vi "Com_SECS Equipment _SECS Packet Write.vi"(8 "error in":errorcluster, 9 "Timeout":i32=1000, 10 "SECS Packet":T1, 11 "Buffer Data In":T5) -> (0 "error out":errorcluster, 3 "Buffer Data Out":T5)   [LabVIEW 2016]
uses:
  Data Def/Com_SECS Equipment _Buffer Data.ctl
  Data Def/Com_SECS Equipment _Connection Setting.ctl
  Data Def/Com_SECS Equipment _Timeout Setting.ctl
  Data Def/Com_SECS Equipment _SECS Packet.ctl
  Data Def/Com_SECS Equipment _Message Type.ctl
  Data Def/Com_SECS Equipment _Protocol Type.ctl
  Data Def/Com_SECS Equipment _Stream Type.ctl
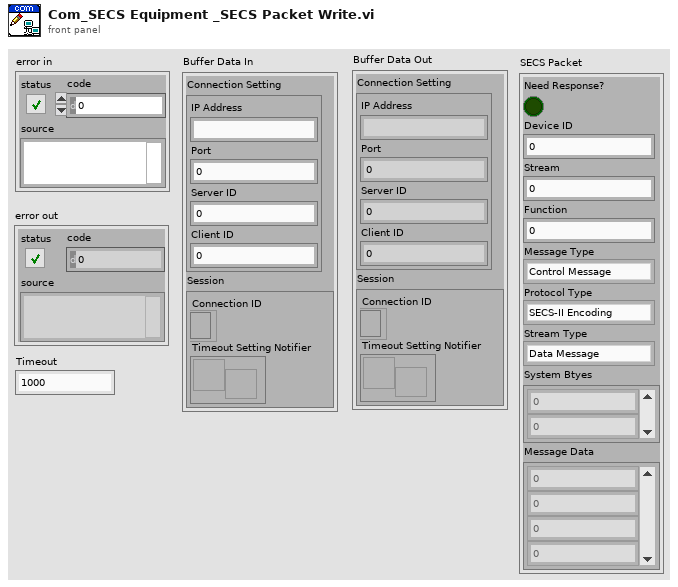
[diagram p1: front panel]
types:
  T1 = typedef "Com_SECS Equipment _SECS Packet.ctl" = cluster{"Need Response?":bool, "Device ID":u16, "Stream":u8, "Function":u8, "Message Type":T2, "Protocol Type":T3, "Stream Type":T4, "System Btyes":u8[], "Message Data":u8[]}
  T2 = typedef "Com_SECS Equipment _Message Type.ctl" = enum16{"Control Message", "Data Message"}
  T3 = typedef "Com_SECS Equipment _Protocol Type.ctl" = enum16{"SECS-II Encoding", "Reserved"}
  T4 = typedef "Com_SECS Equipment _Stream Type.ctl" = enum16{"Data Message", "Select.req", "Select.rsp", "Deselect.req", "Deselect.rsp", "Linktest.req", "Linktest.rsp", "Reject.req", "Separate.req", "Reserve"}
  T5 = typedef "Com_SECS Equipment _Buffer Data.ctl" = cluster{"Connection Setting":T6, "Session":cluster{"Connection ID":refnum<k5>, "Timeout Setting Notifier":refnum<notifier>}}
  T6 = typedef "Com_SECS Equipment _Connection Setting.ctl" = cluster{"IP Address":string, "Port":u16, "Server ID":u16, "Client ID":u16}
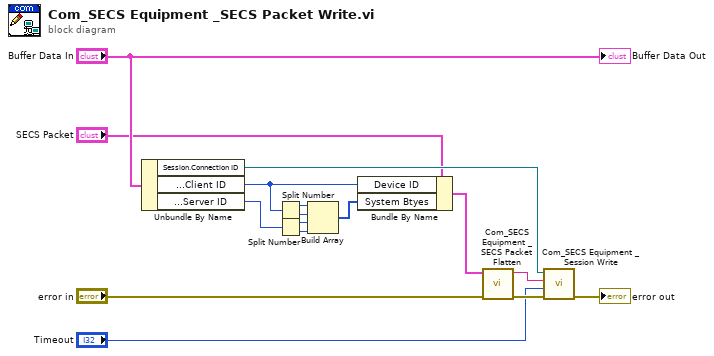
[diagram p0: block diagram]
diagram:
  n1 = Unbundle By Name("Buffer Data In") -> ("Session.Connection ID"=w3:refnum<k5>, "Connection Setting.Client ID"=w11:u16, "Connection Setting.Server ID"=w10:u16)
  n2 = Split Number(x=w11) -> (hi(x)=w9:u8, lo(x)=w8:u8)
  n3 = Split Number(x=w10) -> (hi(x)=w7:u8, lo(x)=w6:u8)
  n4 = Build Array(w9, w8, w7, w6) -> (w5:u8[])
  n5 = Bundle By Name(cluster="SECS Packet", "Device ID"=w11, "System Btyes"=w5) -> (w1:T1)
  n6 = call "Com_SECS Equipment _SECS Packet Flatten.vi"("error in"="error in", "SECS Packet"=w1) -> ("error out"=w15:errorcluster, "Data"=w14:string)  [unwired: 8 in]
  n7 = call "Com_SECS Equipment _Session Write.vi"("error in"=w15, "Timeout(100)"="Timeout", "Write Data"=w14, "Session In"=w3) -> ("error out"=→"error out":errorcluster)  [unwired: 6 in, 1 out]
  "Buffer Data Out" <- "Buffer Data In"
